vi "Pick&Place Tester.vi"() -> ()   [LabVIEW 2017]
uses:
  Shared Components/Gantry Class/Type Definitions/Virtual Modes.ctl
  Shared Components/Gantry Class/Type Definitions/Init_Modes.ctl
  Shared Components/Config Manager Class/Type Definitions/Camera Enum.ctl
  Shared Components/Gantry Class/Gantry Class.lvclass
  Shared Components/Vec3d Class/Vec3d Class.lvclass
panel:
  in  "Virtual Mode":T1=enum."Virtual"
  in  "stop":bool
  out "Image":T2(plugin-control)
  out "error out":errorcluster
  in  "Config Folder":path=path "C:/Users/simra/Desktop/Research/Gantry Purdue/pixel-gantry-control/Config"
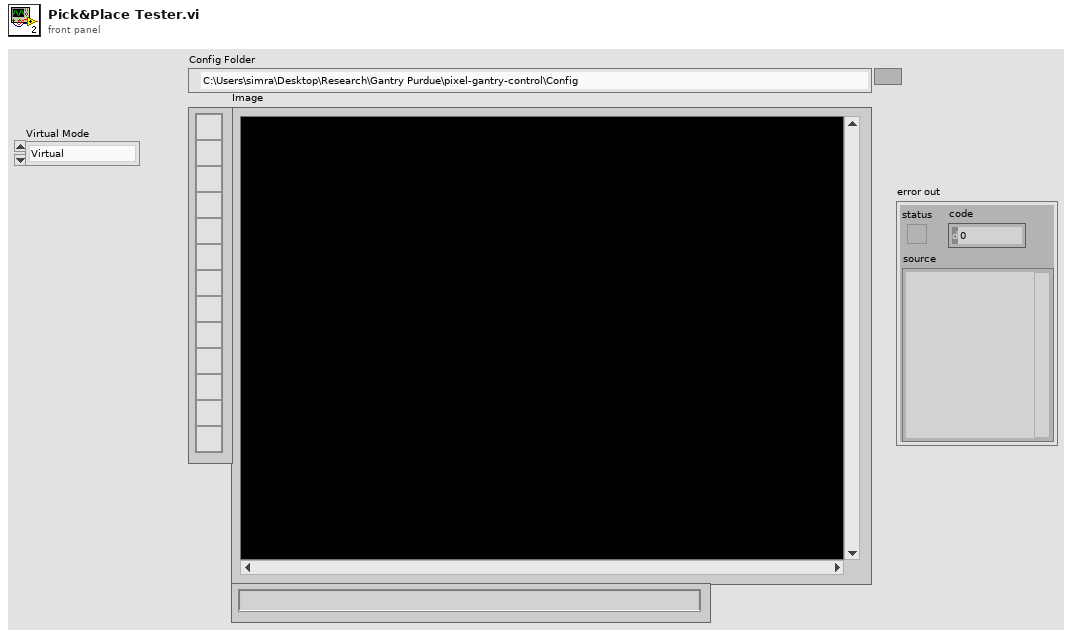
[diagram p1: front panel]
types:
  T1 = typedef "Virtual Modes.ctl" = enum16{"Nonvirtual", "Pseudovirtual", "Virtual"}
  T2 = typedef "IMAQ Image.ctl" = refnum<image>
  T3 = typedef "Camera Enum.ctl" = enum16{"GANTRY HEAD", "NEEDLE CALIBRATION X", "NEEDLE CALIBRATION Y", "STAND CAMERA", "SIMRAN WEBCAM"}
  T4 = typedef "Init_Modes.ctl" = enum16{"Full", "Robot Only", "Dispenser Only", "Cameras Only", "Robot and Cameras", "Robot and Cameras and Dispenser", "Manifold Only"}
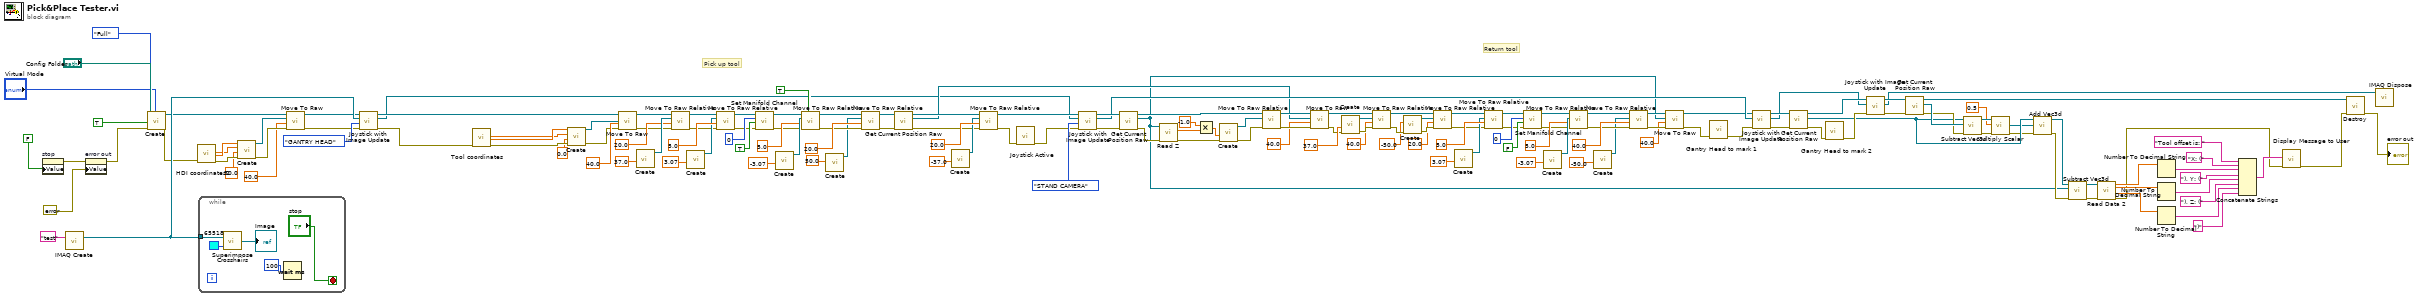
[diagram p0: block diagram]
diagram:
  # "Return tool"
  # "Pick up tool"
  n1 = property on="stop" class="Bool (strict)"("Value"=FALSE) -> (error out=w151:errorcluster)  [unwired: 2 in, 1 out]
  n2 = call "IMAQ Create"("Image Name"="test") -> ("New Image"=w14:T2)  [unwired: 4 in, 1 out]
  n3 = property on="error out" class="Clust (strict)"(error in=w151, "Value"=errorcluster {"status"=FALSE, "code"=0, "source"=""} ("error in (no error)")) -> (error out=w150:errorcluster)  [unwired: 1 in, 1 out]
  n4 = call "Create.vi"("Virtual Mode"="Virtual Mode", "error in"=w150, "HOME?"=TRUE, "Config Folder"="Config Folder", "Init Mode"=Init_Modes."Full") -> ("error out"=w6:errorcluster, "Gantry out"=w4:refnum<class "Gantry Class.lvclass">)  [unwired: 5 in]
  n5 = call "HDI coordinates2"("error in (no error)"=w6) -> ("Y"=w10:dbl, "X"=w11:dbl, "error out"=w9:errorcluster)  [unwired: 15 in, 1 out]
  n6 = while {
    tunnel: w14 -> [w160]
    stop <- "stop" stop-if-true
    n7 = call "Superimpose Crosshairs.vi"("Grid Line Color"=u32 65518, "Refnum in"=w160) -> ("Refnum out"=→"Image":T2)
    n8 = Wait (ms)(milliseconds to wait=u32 100) -> ()  [unwired: 1 out]
  }
  n9 = call "Create.vi"("error in"=w9, "Z"=30.0, "Y"=w10, "X"=w11) -> ("error out"=w2:errorcluster, "Vec3d Class out"=w5:refnum<class "Vec3d Class.lvclass">)  [unwired: 6 in]
  n10 = call-dynamic "Move To Raw.vi"("error in"=w2, "Speed"=40.0, "Destination"=w5, "Gantry in"=w4) -> ("error out"=w7:errorcluster, "Gantry out"=w3:refnum<class "Gantry Class.lvclass">)  [unwired: 6 in]
  n11 = call-dynamic "Joystick with Image Update.vi"("error in (no error)"=w7, "Camera Name"=Camera_Enum."GANTRY HEAD", "Image In"=w14, "Gantry Class in"=w3) -> ("error out"=w15:errorcluster, "Image Out"=w13:T2, "Gantry Class out"=w16:refnum<class "Gantry Class.lvclass">)  [unwired: 5 in]
  n12 = call "Tool coordinates"("error in (no error)"=w15) -> ("Y"=w145:dbl, "X"=w146:dbl, "error out"=w142:errorcluster)  [unwired: 15 in, 1 out]
  n13 = call "Create.vi"("error in"=w142, "Z"=0.0, "Y"=w145, "X"=w146) -> ("error out"=w143:errorcluster, "Vec3d Class out"=w70:refnum<class "Vec3d Class.lvclass">)  [unwired: 6 in]
  n14 = call-dynamic "Move To Raw.vi"("error in"=w143, "Speed"=40.0, "Destination"=w70, "Gantry in"=w16) -> ("error out"=w124:errorcluster, "Gantry out"=w133:refnum<class "Gantry Class.lvclass">)  [unwired: 6 in]
  n15 = call "Create.vi"("Z"=37.0) -> ("Vec3d Class out"=w135:refnum<class "Vec3d Class.lvclass">)  [unwired: 9 in, 1 out]
  n16 = call-dynamic "Move To Raw Relative.vi"("Speed(mm/s)"=20.0, "Delta"=w135, "Gantry in"=w133) -> ("Gantry out"=w126:refnum<class "Gantry Class.lvclass">)  [unwired: 7 in, 1 out]
  n17 = call "Create.vi"("Z"=3.07) -> ("Vec3d Class out"=w127:refnum<class "Vec3d Class.lvclass">)  [unwired: 9 in, 1 out]
  n18 = call-dynamic "Move To Raw Relative.vi"("error in"=w124, "Speed(mm/s)"=5.0, "Delta"=w127, "Gantry in"=w126) -> ("error out"=w123:errorcluster, "Gantry out"=w125:refnum<class "Gantry Class.lvclass">)  [unwired: 6 in]
  n19 = call-dynamic "Set Manifold Channel.vi"("error in"=w123, "On/Off"=TRUE, "Manifold Channel"=0, "Gantry in"=w125) -> ("error out"=w118:errorcluster, "Gantry out"=w119:refnum<class "Gantry Class.lvclass">)  [unwired: 6 in]
  n20 = call "Create.vi"("Z"=-3.07) -> ("Vec3d Class out"=w121:refnum<class "Vec3d Class.lvclass">)  [unwired: 9 in, 1 out]
  n21 = call-dynamic "Move To Raw Relative.vi"("Wait?"=TRUE, "error in"=w118, "Speed(mm/s)"=5.0, "Delta"=w121, "Gantry in"=w119) -> ("error out"=w114:errorcluster, "Gantry out"=w115:refnum<class "Gantry Class.lvclass">)  [unwired: 5 in]
  n22 = call "Create.vi"("Y"=50.0 ("Z")) -> ("Vec3d Class out"=w113:refnum<class "Vec3d Class.lvclass">)  [unwired: 9 in, 1 out]
  n23 = call-dynamic "Move To Raw Relative.vi"("error in"=w114, "Speed(mm/s)"=20.0, "Delta"=w113, "Gantry in"=w115) -> ("error out"=w57:errorcluster, "Gantry out"=w59:refnum<class "Gantry Class.lvclass">)  [unwired: 6 in]
  n24 = call-dynamic "Get Current Position Raw.vi"("error in"=w57, "Gantry in"=w59) -> ("error out"=w56:errorcluster, "Vec3d Class out"=w54:refnum<class "Vec3d Class.lvclass">, "Gantry out"=w58:refnum<class "Gantry Class.lvclass">)  [unwired: 7 in]
  n25 = call "Create.vi"("Z"=-37.0) -> ("Vec3d Class out"=w109:refnum<class "Vec3d Class.lvclass">)  [unwired: 9 in, 1 out]
  n26 = call-dynamic "Move To Raw Relative.vi"("error in"=w56, "Speed(mm/s)"=20.0, "Delta"=w109, "Gantry in"=w58) -> ("error out"=w107:errorcluster, "Gantry out"=w108:refnum<class "Gantry Class.lvclass">)  [unwired: 6 in]
  n27 = call "Joystick Active"("error in (no error)"=w107) -> ("error out"=w106:errorcluster)  [unwired: 17 in, 1 out]
  n28 = call-dynamic "Joystick with Image Update.vi"("error in (no error)"=w106, "Camera Name"=Camera_Enum."STAND CAMERA", "Image In"=w13, "Gantry Class in"=w108) -> ("error out"=w138:errorcluster, "Image Out"=w105:T2, "Gantry Class out"=w139:refnum<class "Gantry Class.lvclass">)  [unwired: 5 in]
  n29 = call-dynamic "Get Current Position Raw.vi"("error in"=w138, "Gantry in"=w139) -> ("error out"=w69:errorcluster, "Vec3d Class out"=w18:refnum<class "Vec3d Class.lvclass">, "Gantry out"=w66:refnum<class "Gantry Class.lvclass">)  [unwired: 7 in]
  n30 = call-dynamic "Read Z.vi"("error in (no error)"=w69, "Vec3d Class in"=w18) -> ("error out"=w65:errorcluster, "Z"=w68:dbl)  [unwired: 7 in, 1 out]
  n31 = Multiply(x=-1.0, y=w68) -> (x*y=w64:dbl)
  n32 = call "Create.vi"("error in"=w65, "Z"=w64) -> ("error out"=w62:errorcluster, "Vec3d Class out"=w63:refnum<class "Vec3d Class.lvclass">)  [unwired: 8 in]
  n33 = call-dynamic "Move To Raw Relative.vi"("error in"=w62, "Delta"=w63, "Gantry in"=w66) -> ("error out"=w61:errorcluster, "Gantry out"=w60:refnum<class "Gantry Class.lvclass">)  [unwired: 7 in]
  n34 = call-dynamic "Move To Raw.vi"("error in"=w61, "Speed"=40.0, "Destination"=w54, "Gantry in"=w60) -> ("error out"=w50:errorcluster, "Gantry out"=w53:refnum<class "Gantry Class.lvclass">)  [unwired: 6 in]
  n35 = call "Create.vi"("error in"=w50, "Z"=37.0) -> ("error out"=w49:errorcluster, "Vec3d Class out"=w52:refnum<class "Vec3d Class.lvclass">)  [unwired: 8 in]
  n36 = call-dynamic "Move To Raw Relative.vi"("error in"=w49, "Speed(mm/s)"=40.0, "Delta"=w52, "Gantry in"=w53) -> ("error out"=w44:errorcluster, "Gantry out"=w45:refnum<class "Gantry Class.lvclass">)  [unwired: 6 in]
  n37 = call "Create.vi"("error in"=w44, "Y"=-50.0) -> ("error out"=w47:errorcluster, "Vec3d Class out"=w17:refnum<class "Vec3d Class.lvclass">)  [unwired: 8 in]
  n38 = call-dynamic "Move To Raw Relative.vi"("error in"=w47, "Speed(mm/s)"=20.0, "Delta"=w17, "Gantry in"=w45) -> ("error out"=w25:errorcluster, "Gantry out"=w26:refnum<class "Gantry Class.lvclass">)  [unwired: 6 in]
  n39 = call "Create.vi"("Z"=3.07) -> ("Vec3d Class out"=w38:refnum<class "Vec3d Class.lvclass">)  [unwired: 9 in, 1 out]
  n40 = call-dynamic "Move To Raw Relative.vi"("error in"=w25, "Speed(mm/s)"=5.0, "Delta"=w38, "Gantry in"=w26) -> ("error out"=w36:errorcluster, "Gantry out"=w37:refnum<class "Gantry Class.lvclass">)  [unwired: 6 in]
  n41 = call-dynamic "Set Manifold Channel.vi"("error in"=w36, "On/Off"=FALSE, "Manifold Channel"=0, "Gantry in"=w37) -> ("error out"=w31:errorcluster, "Gantry out"=w32:refnum<class "Gantry Class.lvclass">)  [unwired: 6 in]
  n42 = call "Create.vi"("Z"=-3.07) -> ("Vec3d Class out"=w34:refnum<class "Vec3d Class.lvclass">)  [unwired: 9 in, 1 out]
  n43 = call-dynamic "Move To Raw Relative.vi"("error in"=w31, "Speed(mm/s)"=5.0, "Delta"=w34, "Gantry in"=w32) -> ("error out"=w28:errorcluster, "Gantry out"=w29:refnum<class "Gantry Class.lvclass">)  [unwired: 6 in]
  n44 = call "Create.vi"("Z"=-50.0) -> ("Vec3d Class out"=w27:refnum<class "Vec3d Class.lvclass">)  [unwired: 9 in, 1 out]
  n45 = call-dynamic "Move To Raw Relative.vi"("error in"=w28, "Speed(mm/s)"=40.0, "Delta"=w27, "Gantry in"=w29) -> ("error out"=w22:errorcluster, "Gantry out"=w23:refnum<class "Gantry Class.lvclass">)  [unwired: 6 in]
  n46 = call-dynamic "Move To Raw.vi"("error in"=w22, "Speed"=40.0, "Destination"=w18, "Gantry in"=w23) -> ("error out"=w19:errorcluster, "Gantry out"=w20:refnum<class "Gantry Class.lvclass">)  [unwired: 6 in]
  n47 = call "Gantry Head to mark 1"("error in (no error)"=w19) -> ("error out"=w147:errorcluster)  [unwired: 9 in, 1 out]
  n48 = call-dynamic "Joystick with Image Update.vi"("error in (no error)"=w147, "Image In"=w105, "Gantry Class in"=w20) -> ("error out"=w152:errorcluster, "Image Out"=w79:T2, "Gantry Class out"=w153:refnum<class "Gantry Class.lvclass">)  [unwired: 6 in]
  n49 = call-dynamic "Get Current Position Raw.vi"("error in"=w152, "Gantry in"=w153) -> ("error out"=w100:errorcluster, "Vec3d Class out"=w94:refnum<class "Vec3d Class.lvclass">, "Gantry out"=w101:refnum<class "Gantry Class.lvclass">)  [unwired: 7 in]
  n50 = call "Gantry Head to mark 2"("error in (no error)"=w100) -> ("error out"=w102:errorcluster)  [unwired: 9 in, 1 out]
  n51 = call-dynamic "Joystick with Image Update.vi"("error in (no error)"=w102, "Image In"=w79, "Gantry Class in"=w101) -> ("error out"=w103:errorcluster, "Image Out"=w78:T2, "Gantry Class out"=w104:refnum<class "Gantry Class.lvclass">)  [unwired: 6 in]
  n52 = call-dynamic "Get Current Position Raw.vi"("error in"=w103, "Gantry in"=w104) -> ("error out"=w98:errorcluster, "Vec3d Class out"=w99:refnum<class "Vec3d Class.lvclass">, "Gantry out"=w90:refnum<class "Gantry Class.lvclass">)  [unwired: 7 in]
  n53 = call "Subtract Vec3d.vi"("error in (no error)"=w98, "Vec3d in 2"=w99, "Vec3d in 1"=w94) -> ("error out"=w96:errorcluster, "Vec3d Class out"=w97:refnum<class "Vec3d Class.lvclass">)  [unwired: 7 in]
  n54 = call-dynamic "Multiply Scalar.vi"("error in"=w96, "Scale"=0.5, "Vec3d in"=w97) -> ("error out"=w92:errorcluster, "Vec3d out"=w93:refnum<class "Vec3d Class.lvclass">)  [unwired: 7 in]
  n55 = call-dynamic "Add Vec3d.vi"("error in (no error)"=w92, 10:"Vec3d Class in"=w93, 11:"Vec3d Class in"=w94) -> ("error out"=w89:errorcluster, "Vec3d Class out"=w91:refnum<class "Vec3d Class.lvclass">)  [unwired: 7 in]
  n56 = call "Subtract Vec3d.vi"("error in (no error)"=w89, "Vec3d in 2"=w18, "Vec3d in 1"=w91) -> ("error out"=w87:errorcluster, "Vec3d Class out"=w88:refnum<class "Vec3d Class.lvclass">)  [unwired: 7 in]
  n57 = call-dynamic "Read Data 2.vi"("error in"=w87, "Vec3d in"=w88) -> ("error out"=w81:errorcluster, "Z"=w84:dbl, "Y"=w85:dbl, "X"=w86:dbl)  [unwired: 6 in]
  n58 = Number To Decimal String(number=w85) -> (decimal integer string=w77:string)  [unwired: 1 in]
  n59 = Number To Decimal String(number=w86) -> (decimal integer string=w83:string)  [unwired: 1 in]
  n60 = Number To Decimal String(number=w84) -> (decimal integer string=w73:string)  [unwired: 1 in]
  n61 = Concatenate Strings("Tool offset is: " ("string"), "X: (" ("string"), w83, "), Y: (" ("string"), w77, "), Z: (" ("string"), w73, ")" ("string")) -> (w82:string)
  n62 = call "Display Message to User"("error in (no error)"=w81, "Message"=w82) -> ("error out"=w80:errorcluster)  [unwired: 8 in, 1 out]
  n63 = call "Destroy.vi"("error in"=w80, "Gantry Class in"=w90) -> ("error out"=→"error out":errorcluster)  [unwired: 9 in]
  n64 = call "IMAQ Dispose"("Image"=w78) -> ()  [unwired: 5 in, 1 out]
